vi "Actor Core.vi"(8 "Error In":errorcluster, 11 "CS++RTSystemHealthActor in":refnum<class "CS++RTSystemHealthActor.lvclass">) -> (0 "Error Out":errorcluster, 3 "Actor out":refnum<class "Actor.lvclass">)   [LabVIEW 2015, in "CS++RTSystemHealth.lvlib" / "CS++RTSystemHealthActor.lvclass"]
doc: "Publish system status and disc information to statically bound shared variables. \n\n(<B>Filename</B>: Actor Framework.lvlib:Actor.lvclass:Actor Core.vi)\n\nReceives messages to the actor, reacts to them, and initiates any error handling that may shut the actor down.\n\nDescendant classes may override this VI to append parallel tasks for the actor to complete while it handles messages. Overrides use the Call Parent Method node."
uses:
  CS++RTSystemHealthActor.lvclass
  <vilib>/ActorFramework/Actor/Actor.lvclass
  CS++RTSystemHealthActor.lvclass/CS++RTSystemHealthActor.ctl
  <vilib>/ActorFramework/Actor/Actor.lvclass/Actor.ctl
  CSPP_Core/Libraries/Base/Severity.ctl
  <vilib>/ActorFramework/Report Error Msg/Report Error Msg.lvclass/Report Error Msg.ctl
  <vilib>/ActorFramework/Message Enqueuer/Message Enqueuer.lvclass/Message Enqueuer.ctl
  <vilib>/ActorFramework/Message Enqueuer/Enqueue.vi
  <vilib>/nisyscfg/Close (System).vi
  <vilib>/ActorFramework/Message Priority Queue/Priority Enqueue.vi
  <vilib>/ActorFramework/Report Error Msg/Report Error Msg.lvclass
  <vilib>/nisyscfg/nisyscfg.lvlib
  <resource>/objmgr/nisysapi.rc
  CSPP_Core/Libraries/Utilities/CS++Utilities.lvlib
  CSPP_Core/Libraries/Base/CS++Base.lvlib
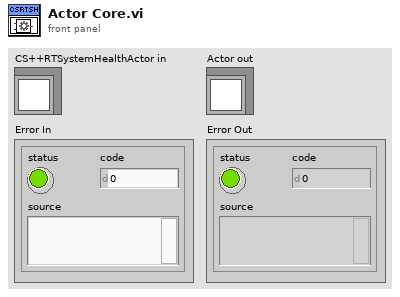
[diagram p1: front panel]
types:
  T1 = typedef "CS++Base.lvlib/Severity.ctl" = enum16{"emergency", "alert", "critical", "error", "warning", "notice", "info", "debug"}
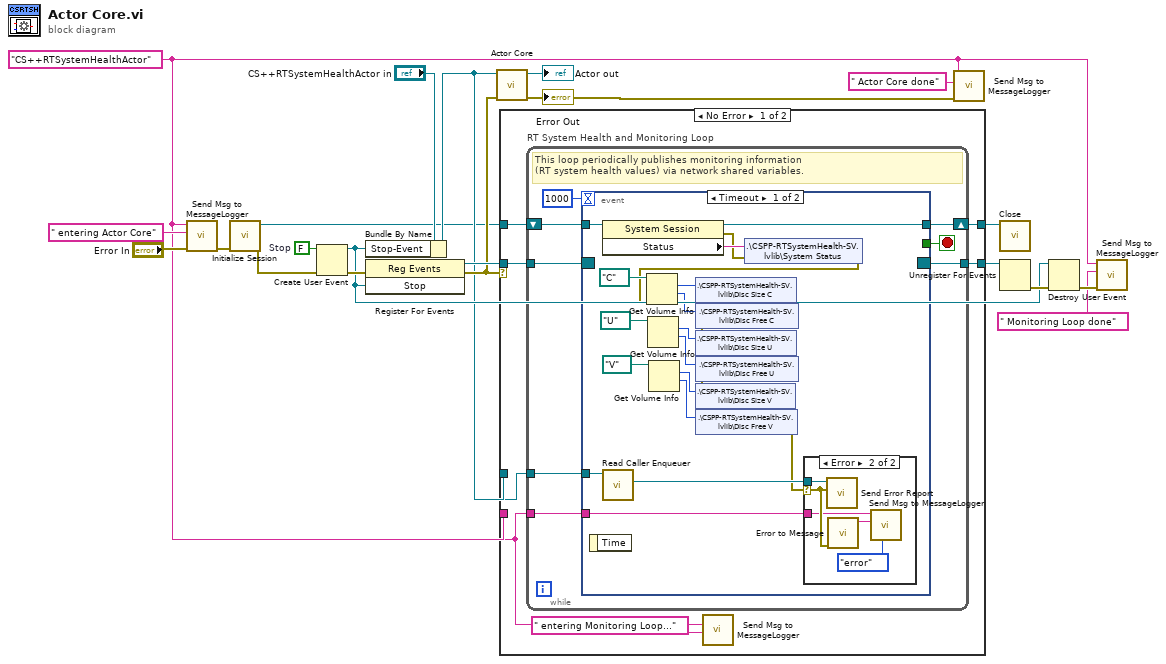
[diagram p0: block diagram]
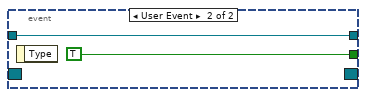
[diagram p3: hidden frame]
diagram:
  w1 = "CS++RTSystemHealthActor" ("String to write")
  w19 = FALSE  # Stop
  n1 = call "Send Msg to MessageLogger.vi"("Error In"="Error In", "Message Content"=" entering Actor Core" ("String to write"), "Message Tag"=w1) -> ("Error Out"=w7:errorcluster)  [unwired: 8 in]
  n2 = call <vilib>:"Initialize Session.vi"("error in (no error)"=w7) -> ("error out"=w16:errorcluster, "Session out"=w9:refnum<k21>)  [unwired: 9 in]
  n3 = Create User Event(user event datatype=w19, error in=w16) -> (user event=w12:refnum<user-event>, error out=w18:errorcluster)
  n4 = Bundle By Name(cluster="CS++RTSystemHealthActor in", "Stop-Event"=w12) -> (w10:refnum<class "CS++RTSystemHealthActor.lvclass">)
  n5 = register-events(error in=w18, w12) -> (reference out=w17:refnum<event-registration>, error out=w15:errorcluster)  [unwired: 1 in]
  n6 = call-parent "Actor Core.vi"("error in"=w15, "Actor in"=w10) -> ("error out"=w4:errorcluster, "Actor out"=→"Actor out":refnum<class "Actor.lvclass">)  [unwired: 8 in]
  "Error Out" <- w4
  n7 = case shown="No Error" w15 {
    tunnel: w9 -> [w28 w69]
    tunnel: [w27 w69] -> w20
    tunnel: w17 -> [w26 w68]
    tunnel: [w25 w68] -> w14
    tunnel: w10 -> [w24 _]
    tunnel: w1 -> [w22 _]
    frame No Error {
      n8 = while "RT System Health and Monitoring Loop" {
        shift-right: [w35] -> w27
        shift-left: w28 -> [w36]
        tunnel: w26 -> [w33]
        tunnel: [w32] -> w25
        tunnel: w24 -> [w30]
        tunnel: w22 -> [w29]
        stop <- w31 stop-if-true
        # "This loop periodically publishes monitoring information\n(RT system health values) via network shared variables."
        n9 = event shown="[0] Timeout" {
          selector: w33 -> [_ _]
          dyn-events: [_ _] -> w32
          timeout: 1000 -> [_ _]
          tunnel: w36 -> [w57 w67]
          tunnel: [w56 w67] -> w35
          tunnel: [_ TRUE] -> w31
          tunnel: w30 -> [w59 _]
          tunnel: w29 -> [w48 _]
          event Timeout {
            n10 = event-data() -> ()  [unwired: 1 in, 1 out]
            n11 = property class="System Session"(reference=w57) -> (reference out=w56:refnum<k21>, error out=w54:errorcluster, "Status"=w55:string)  [unwired: 1 in]
            n12 = call <vilib>:"Read Caller Enqueuer.vi"("Actor"=w59) -> ("Caller Enqueuer"=w58:refnum<class "Message Enqueuer.lvclass">)  [unwired: 10 in]
            n13 = Get Volume Info(11:path "U:/" ("path")) -> (1:w47:i64, 2:w46:i64)  [unwired: 1 in, 4 out]
            n14 = Get Volume Info(11:path "V:/" ("path")) -> (1:w42:i64, 2:w43:i64)  [unwired: 1 in, 4 out]
            n15 = shared-variable ".\\CSPP-RTSystemHealth-SV.lvlib\\System Status"(w55, error in=w54) -> (error out=w53:errorcluster)
            n16 = Get Volume Info(8:w53, 11:path "C:/" ("path")) -> (0:w51:errorcluster, 1:w50:i64, 2:w52:i64)  [unwired: 3 out]
            n17 = shared-variable ".\\CSPP-RTSystemHealth-SV.lvlib\\Disc Size C"(w52, error in=w51) -> (error out=w49:errorcluster)
            n18 = shared-variable ".\\CSPP-RTSystemHealth-SV.lvlib\\Disc Free C"(w50, error in=w49) -> (error out=w41:errorcluster)
            n19 = shared-variable ".\\CSPP-RTSystemHealth-SV.lvlib\\Disc Size U"(w46, error in=w41) -> (error out=w40:errorcluster)
            n20 = shared-variable ".\\CSPP-RTSystemHealth-SV.lvlib\\Disc Free U"(w47, error in=w40) -> (error out=w37:errorcluster)
            n21 = shared-variable ".\\CSPP-RTSystemHealth-SV.lvlib\\Disc Size V"(w43, error in=w37) -> (error out=w39:errorcluster)
            n22 = shared-variable ".\\CSPP-RTSystemHealth-SV.lvlib\\Disc Free V"(w42, error in=w39) -> (error out=w38:errorcluster)
            n23 = case shown="Error" w38 {
              selector: w38 -> [_ w64]
              tunnel: w58 -> [_ w65]
              tunnel: w48 -> [_ w62]
              frame No Error {
              }
              frame Error {
                n24 = call <vilib>:"Send Error Report.vi"("Error From Sender"=w64, "Message Enqueuer"=w65) -> ()  [unwired: 9 in, 1 out]
                n25 = call "Error to Message.vi"("Error In"=w64) -> ("Error Message"=w63:string)  [unwired: 9 in, 1 out]
                n26 = call "Send Msg to MessageLogger.vi"("Severity Code (info)"=Severity."error", "Message Content"=w63, "Message Tag"=w62) -> ()  [unwired: 8 in, 1 out]
              }
            }
          }
          event User Event {
            n27 = event-data() -> ()  [unwired: 1 in, 1 out]
          }
        }
      }
      n28 = call "Send Msg to MessageLogger.vi"("Message Content"=" entering Monitoring Loop..." ("String to write"), "Message Tag"=w22) -> ()  [unwired: 9 in, 1 out]
    }
    frame Error {
    }
  }
  n29 = call "Send Msg to MessageLogger.vi"("Error In"=w4, "Message Content"=" Actor Core done" ("String to write"), "Message Tag"=w1) -> ()  [unwired: 8 in, 1 out]
  n30 = call-poly <vilib>:"Close.vi"("Session in"=w20) -> ()  [unwired: 10 in, 1 out]
  n31 = Unregister For Events(event registration refnum=w14) -> (error out=w13:errorcluster)  [unwired: 1 in]
  n32 = Destroy User Event(user event=w12, error in=w13) -> (error out=w3:errorcluster)
  n33 = call "Send Msg to MessageLogger.vi"("Error In"=w3, "Message Content"=" Monitoring Loop done" ("String to write"), "Message Tag"=w1) -> ()  [unwired: 8 in, 1 out]
